vi "Read Inputs (Batch).vi"(0 "connection ID":refnum<k16>, 1 "address":u32, 2 "port":u16, 9 "timeout ms (1000)":i32=1000, 11 "error in (no error)":errorcluster) -> (4 "connection ID out":refnum<k16>, 6 "received data":string, 8 "Inputs":bool[](array[boolean]), 15 "error out":errorcluster)   [LabVIEW 2016, in "instr.lvlib"]
doc: "Reads all digital states of only input pins and returns them as array. Batch operation."
uses:
  instr.lvlib
  IO State.ctl
panel:
  out "Send String":string
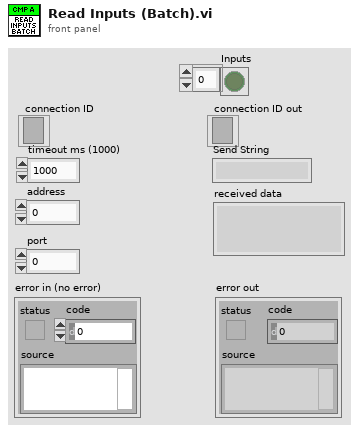
[diagram p1: front panel]
types:
  T1 = typedef "instr.lvlib/IO State.ctl" = u16
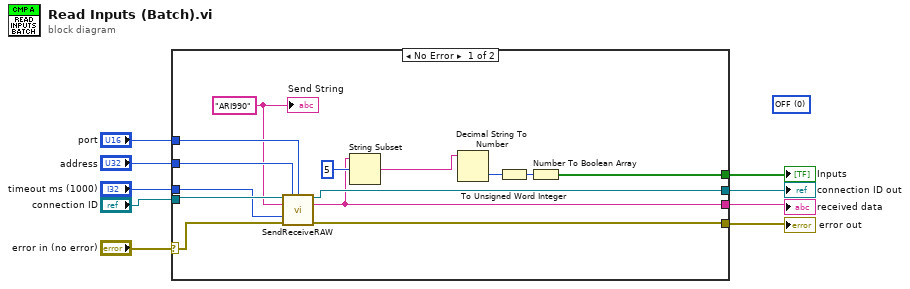
[diagram p0: block diagram]
diagram:
  (unwired) T1 0 items=["OFF", "ON"] ("Relay State")
  n1 = case shown="No Error" "error in (no error)" {
    selector: "error in (no error)" -> [w10 w25]
    tunnel: [w23 w25] -> w9
    tunnel: "timeout ms (1000)" -> [w20 _]
    tunnel: "connection ID" -> [w21 w24]
    tunnel: [w22 w24] -> w5
    tunnel: "address" -> [w19 _]
    tunnel: "port" -> [w18 _]
    tunnel: [w15 _] -> w2
    tunnel: [w12 _] -> w1
    frame No Error {
      w17 = "ARI990" ("data in")
      n2 = call "SendReceiveRAW.vi"("connection ID"=w21, "address"=w19, "port"=w18, "RAW data in"=w17, "timeout ms (1000)"=w20, "error in (no error)"=w10) -> ("connection ID out"=w22:refnum<k16>, "received data"=w15:string, "error out"=w23:errorcluster)  [unwired: 7 in]
      n3 = String Subset(string=w15, offset (0)=5 ("offset")) -> (substring=w11:string)  [unwired: 1 in]
      n4 = Decimal String To Number(string=w11) -> (number=w14:i32)  [unwired: 2 in, 1 out]
      n5 = To Unsigned Word Integer(number=w14) -> (unsigned 16bit integer=w13:u16)
      n6 = Number To Boolean Array(number=w13) -> (Boolean array=w12:bool[])
      "Send String" <- w17
    }
    frame Error {
    }
  }
  "error out" <- w9
  "received data" <- w2
  "connection ID out" <- w5
  "Inputs" <- w1
